vi "Wait For Command.vi"(8 "error in (no error)":errorcluster, 9 "timeout in ms (0)":i32 format="%d ms", 11 "Logging Thread in":refnum<class "Logging Thread.lvclass">) -> (0 "error out":errorcluster, 2 "command":T1={"Command"=enum."Log Plugin State", "Parameters"={"arg1"=0, "arg2"=0}}, 3 "Logging Thread out":refnum<class "Logging Thread.lvclass">)   [LabVIEW 2019, in "DSF Core.lvlib" / "Logging Thread.lvclass"]
uses:
  Logging Thread.lvclass
  Interface/Logging/Command Data.ctl
  Interface/Logging/Command.ctl
  Interface/Logging/Parameters.ctl
  Logging Thread.lvclass/Logging Thread.ctl
  Interface/Interface.lvclass/Interface.ctl
  Interface/Logging/Wait For Logging Command.vi
  Interface/Errors.vi
  Interface/Dispatcher/Command Timeout.vi
  Interface/Read RT FIFO.vi
  Interface/New Interface Error.vi
  <vilib>/NI/Memory Manager/VIs/New Error Cluster.vi
  <vilib>/NI/Memory Manager/VIs/New Error Cluster (512B).vi
  <vilib>/NI/Memory Manager/VIs/Set Error Code.vi
  <vilib>/NI/Memory Manager/VIs/Set Error Status.vi
  <vilib>/NI/Memory Manager/VIs/Set Error Source.vi
  <vilib>/NI/Memory Manager/VIs/Write String to Source.vi
  Interface/Interface Error Info.vi
  VIs/Constants/Constants.vi
  VIs/Constants/Base Error Code.vi
  Interface/Interface Error Offset.vi
  Interface/Logging/Logging Interface.lvclass
  C:/Dev/GitHub/niveristand-data-sharing-framework-custom-device/Core/Classes/Interface/Interface.lvclass
  VIs/VI Name.vi
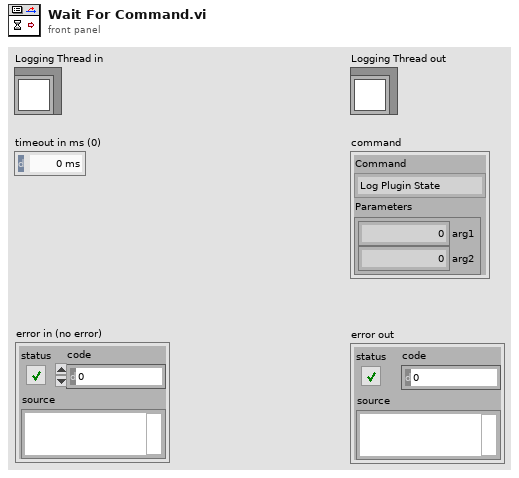
[diagram p1: front panel]
types:
  T1 = typedef "DSF Core.lvlib/Logging Interface.lvclass/Command Data.ctl" = cluster{"Command":T2, "Parameters":T3}
  T2 = typedef "DSF Core.lvlib/Logging Interface.lvclass/Command.ctl" = enum8{"Idle", "Start", "Log Framework State", "Log Plugin State", "Log Dispatcher State", "Shutdown"}
  T3 = typedef "DSF Core.lvlib/Logging Interface.lvclass/Parameters.ctl" = cluster{"arg1":u64, "arg2":u64}
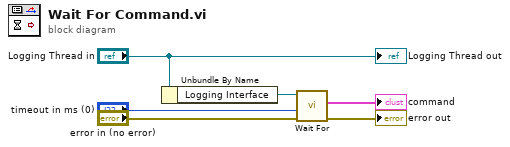
[diagram p0: block diagram]
diagram:
  n1 = Unbundle By Name("Logging Thread in") -> ("Logging Interface"=w3:refnum<class "Logging Interface.lvclass">)
  n2 = call-poly "Wait For.vi"("error in (no error)"="error in (no error)", "timeout in ms (0)"="timeout in ms (0)", "Logging Interface in"=w3) -> ("error out"=→"error out":errorcluster, "command"=→"command":T1)  [unwired: 5 in, 2 out]
  "Logging Thread out" <- "Logging Thread in"
